vi "JW24F14MessageLoop.vi"(8 "Error In":errorcluster, 11 "CommunicationRefs":T1) -> (0 "Error Out":errorcluster)   [LabVIEW 2015]
uses:
  TypeDefs/CommunicationRefs.ctl
  TypeDefs/MessageCluster.ctl
  TypeDefs/JW24F14Settings.ctl
  <vilib>/Utility/inputDevices.llb/joystickAcquire.vi
  <vilib>/Utility/inputDevices.llb/closeJoystick.vi
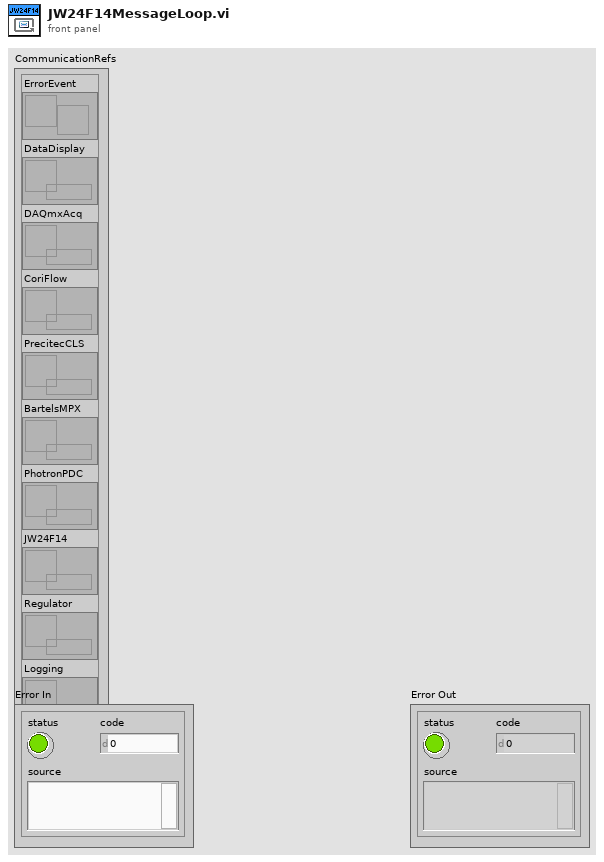
[diagram p1: front panel]
types:
  T1 = typedef "CommunicationRefs.ctl" = cluster{"ErrorEvent":refnum<user-event>, "DataDisplay":refnum<queue>, "DAQmxAcq":refnum<queue>, "CoriFlow":refnum<queue>, "PrecitecCLS":refnum<queue>, "BartelsMPX":refnum<queue>, "PhotronPDC":refnum<queue>, "JW24F14":refnum<queue>, "Regulator":refnum<queue>, "Logging":refnum<queue>}
  T2 = typedef "JW24F14Settings.ctl" = cluster{"Simulate":bool, "device index":i32}
  T3 = cluster{"X axis":i32, "Y axis":i32, "Z axis":i32, "X axis rotation":i32, "Y axis rotation":i32, "Z axis rotation":i32, "U axis":i32, "V axis":i32}
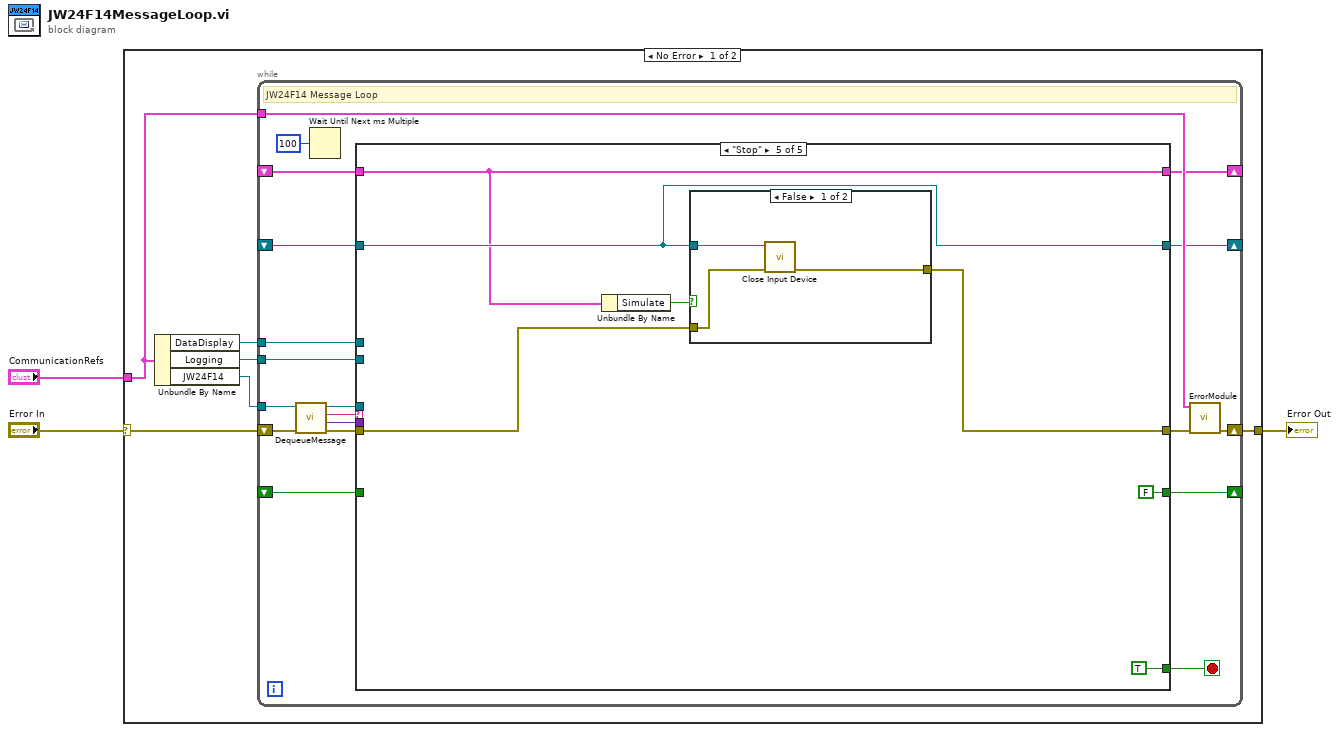
[diagram p0: block diagram]
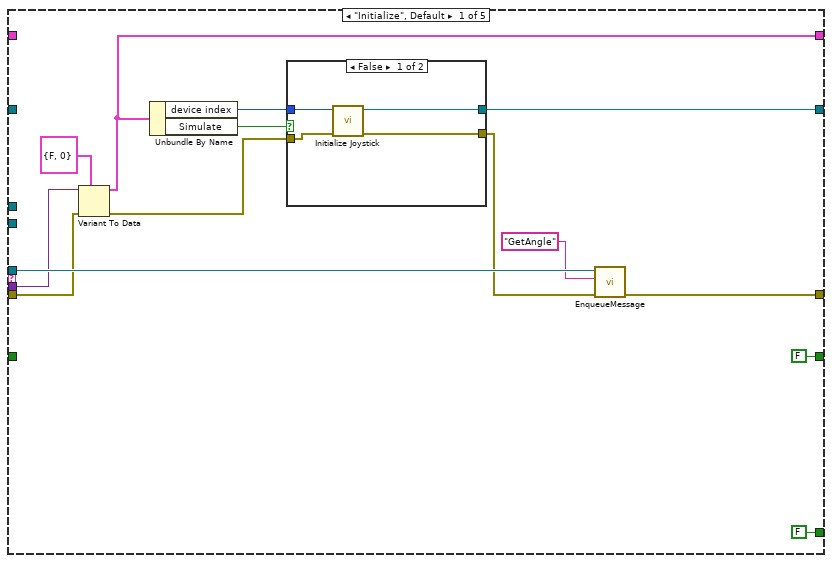
[diagram p2: hidden frame]
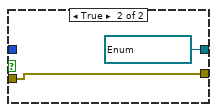
[diagram p3: hidden frame]
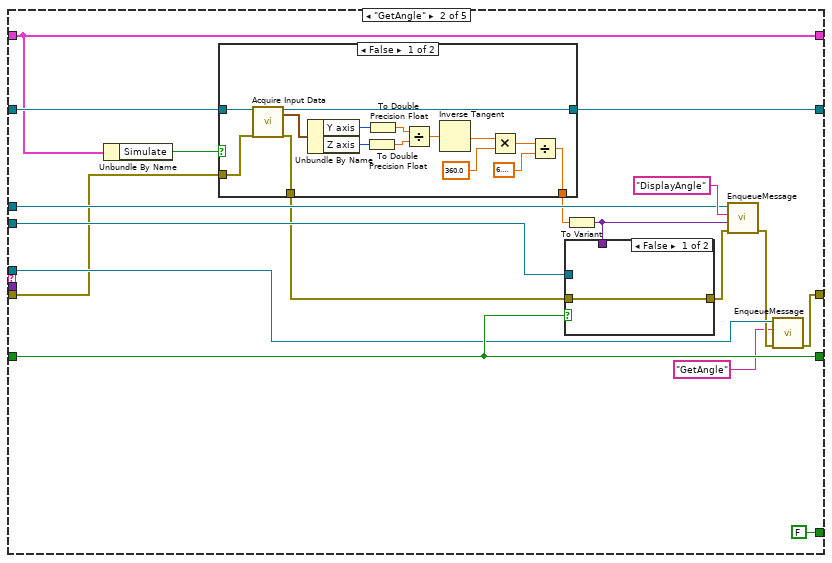
[diagram p4: hidden frame]
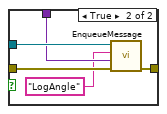
[diagram p5: hidden frame]
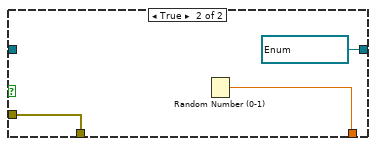
[diagram p6: hidden frame]
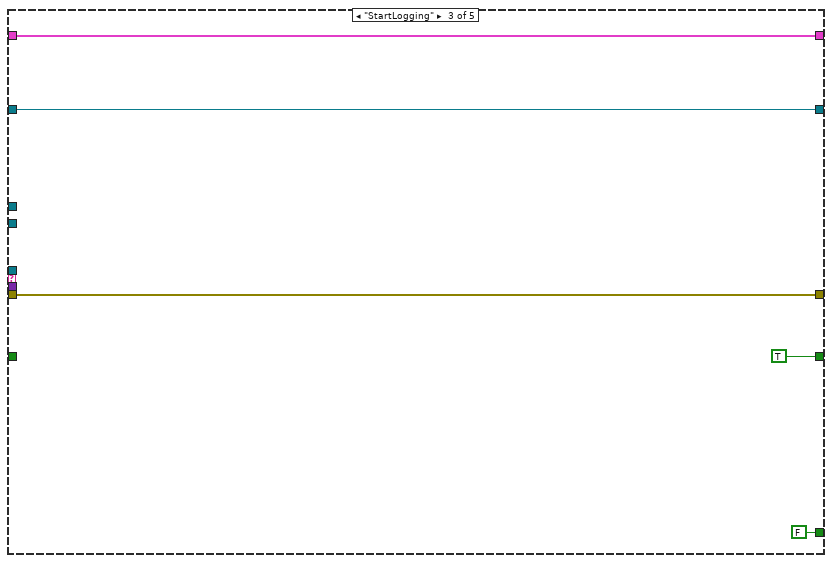
[diagram p7: hidden frame]
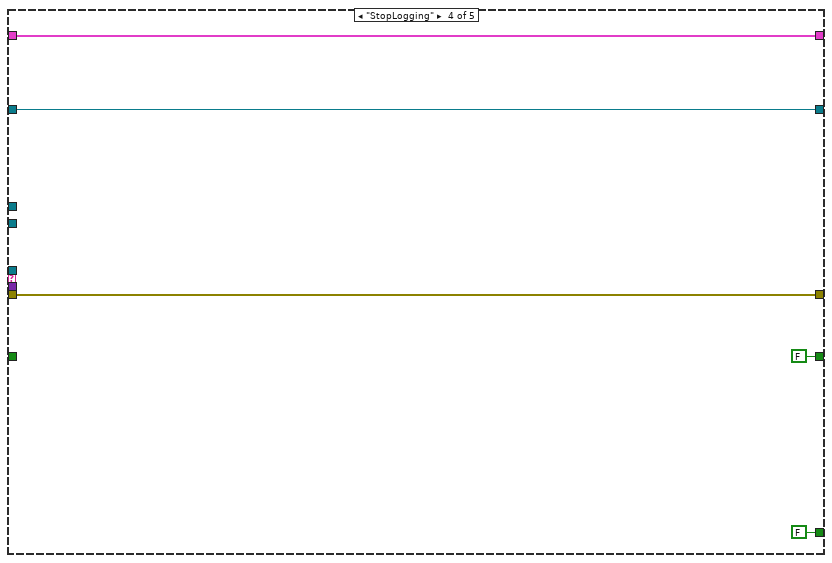
[diagram p8: hidden frame]
diagram:
  n1 = case shown="No Error" "Error In" {
    selector: "Error In" -> [w8 w112]
    tunnel: [w7 w112] -> w2
    tunnel: "CommunicationRefs" -> [w6 _]
    frame No Error {
      n2 = Unbundle By Name(w6) -> ("DataDisplay"=w5:refnum<queue>, "Logging"=w4:refnum<queue>, "JW24F14"=w9:refnum<queue>)
      n3 = while {
        tunnel: w9 -> [w28]
        tunnel: w6 -> [w20]
        shift-right: [w22] -> w7
        shift-left: w8 -> [w27]
        tunnel: w5 -> [w18]
        tunnel: w4 -> [w17]
        shift-right: [w16] -> _
        shift-left: _ -> [w15]
        shift-right: [w14] -> _
        shift-left: _ -> [w13]
        shift-right: [w11] -> _
        shift-left: _ -> [w10]
        stop <- w19 stop-if-true
        # "JW24F14 Message Loop"
        n4 = call "DequeueMessage.vi"("error in (no error)"=w27, "MessageQueue"=w28) -> ("error out"=w23:errorcluster, "MessageData"=w24:variant, "Message"=w25:string, "dupMessageQueue"=w26:refnum<queue>)  [unwired: 6 in]
        n5 = Wait Until Next ms Multiple(millisecond multiple=u32 100) -> ()  [unwired: 1 out]
        n6 = case shown="\"Stop\"" w25 {
          tunnel: w26 -> [w40 w55 _ _ _]
          tunnel: w24 -> [w38 _ _ _ _]
          tunnel: w23 -> [w34 w51 w94 w100 w103]
          tunnel: [w30 w53 w94 w100 w104] -> w21
          tunnel: [FALSE FALSE FALSE FALSE TRUE] -> w19
          tunnel: w18 -> [_ w62 _ _ _]
          tunnel: w17 -> [_ w59 _ _ _]
          tunnel: [FALSE w60 TRUE FALSE FALSE] -> w16
          tunnel: w15 -> [_ w60 _ _ _]
          tunnel: [w32 w64 w92 w97 w105] -> w14
          tunnel: w13 -> [_ w65 w92 w97 w105]
          tunnel: [w29 w49 w91 w96 w102] -> w11
          tunnel: w10 -> [_ w49 w91 w96 w102]
          frame "Initialize", Default {
            n7 = Variant To Data(error in=w34, type=T2 {"Simulate"=FALSE, "device index"=0} ("JW24F14Settings"), Variant=w38) -> (data=w29:T2, error out=w33:errorcluster)
            n8 = Unbundle By Name(w29) -> ("device index"=w35:i32, "Simulate"=w36:bool)
            n9 = case shown="False" w36 {
              tunnel: w35 -> [w46 _]
              tunnel: w33 -> [w45 w48]
              tunnel: [w44 w47] -> w32
              tunnel: [w43 w48] -> w31
              frame False {
                n10 = call <vilib>:"Initialize Joystick.vi"("error in (no error)"=w45, "device index"=w46) -> ("error out"=w43:errorcluster, "device ID"=w44:refnum<k1>)  [unwired: 8 in]
              }
              frame True {
                w47 = refnum<k1> refnum items=["JOYSTICK"] ("device ID")
              }
            }
            n11 = call "EnqueueMessage.vi"("error in (no error)"=w31, "Message"="GetAngle", "MessageQueue"=w40) -> ("error out"=w30:errorcluster)  [unwired: 7 in, 1 out]
          }
          frame "GetAngle" {
            n12 = Unbundle By Name(w49) -> ("Simulate"=w50:bool)
            n13 = case shown="False" w50 {
              tunnel: w65 -> [w87 _]
              tunnel: w51 -> [w86 w89]
              tunnel: [w84 w90] -> w64
              tunnel: [w74 w88] -> w61
              tunnel: [w73 w89] -> w57
              frame False {
                n14 = call-poly <vilib>:"Acquire Input Data.vi"("device ID"=w87, "error in (no error)"=w86) -> ("device ID"=w84:refnum<k1>, "axis info"=w85:T3, "error out"=w73:errorcluster)  [unwired: 13 in, 2 out]
                n15 = Unbundle By Name(w85) -> ("Y axis"=w83:i32, "Z axis"=w82:i32)
                n16 = To Double Precision Float(number=w82) -> (double precision float=w80:dbl)
                n17 = To Double Precision Float(number=w83) -> (double precision float=w81:dbl)
                n18 = Divide(x=w81, y=w80) -> (x/y=w79:dbl)
                n19 = Inverse Tangent(1:w79) -> (0:w78:dbl)
                n20 = Multiply(x=w78, y=360.0) -> (x*y=w76:dbl)
                n21 = Divide(x=w76, y=6.283185307179586) -> (x/y=w74:dbl)
              }
              frame True {
                w90 = refnum<k1> refnum items=["JOYSTICK"] ("device ID")
                n22 = Random Number (0-1)() -> (number: 0 to 1=w88:dbl)
              }
            }
            n23 = To Variant(anything=w61) -> (Variant=w56:variant)
            n24 = case shown="False" w60 {
              tunnel: w59 -> [_ w72]
              tunnel: [w67 w71] -> w58
              tunnel: w57 -> [w67 w70]
              tunnel: w56 -> [_ w69]
              frame False {
              }
              frame True {
                n25 = call "EnqueueMessage.vi"("error in (no error)"=w70, "MessageData"=w69, "Message"="LogAngle", "MessageQueue"=w72) -> ("error out"=w71:errorcluster)  [unwired: 6 in, 1 out]
              }
            }
            n26 = call "EnqueueMessage.vi"("error in (no error)"=w58, "MessageData"=w56, "Message"="DisplayAngle", "MessageQueue"=w62) -> ("error out"=w54:errorcluster)  [unwired: 6 in, 1 out]
            n27 = call "EnqueueMessage.vi"("error in (no error)"=w54, "Message"="GetAngle", "MessageQueue"=w55) -> ("error out"=w53:errorcluster)  [unwired: 7 in, 1 out]
          }
          frame "StartLogging" {
          }
          frame "StopLogging" {
          }
          frame "Stop" {
            n28 = Unbundle By Name(w102) -> ("Simulate"=w101:bool)
            n29 = case shown="False" w101 {
              tunnel: w105 -> [w110 _]
              tunnel: w103 -> [w109 w111]
              tunnel: [w108 w111] -> w104
              frame False {
                n30 = call-poly <vilib>:"Close Input Device.vi"("error in (no error)"=w109, "device ID"=w110) -> ("error out"=w108:errorcluster)  [unwired: 8 in]
              }
              frame True {
              }
            }
          }
        }
        n31 = call "ErrorModule.vi"("Error In"=w21, "CommunicationRefs"=w20) -> ("Error Out"=w22:errorcluster)  [unwired: 9 in]
      }
    }
    frame Error {
    }
  }
  "Error Out" <- w2
